vi "SPWB_Create.vi"(0 "reference in":refnum<class "SPWB.lvclass">, 5 "error in (no error)":errorcluster, 6 "Version #":string, 7 "Application Name":string, 9 "Window Name Index":string, 11 "State Queue":string[](array[string])) -> (14 "reference out":refnum<class "SPWB.lvclass">, 19 "error out":errorcluster)   [LabVIEW 2022 SP3, in "SPWB.lvclass"]
doc: "Constructor."
uses:
  SPWB.lvclass
  C:/Program Files/National Instruments/LabVIEW 2022/vi.lib/addons/_AddQ/G#Object/G#Object.lvclass
  W:/projects/archives/23 Charette AI Group/SPWB/API/Generic Utilities_class/Generic Utilities.lvclass
  API/Registration_class/utils/Registration Type.ctl
  <vilib>/addons/_AddQ/G#Object/G#Object.lvclass
  API/GSwFormDSP_class/GSwFormDSP.lvclass
  API/Generic Utilities_class/Generic Utilities.lvclass
  API/Registration_class/Registration.lvclass
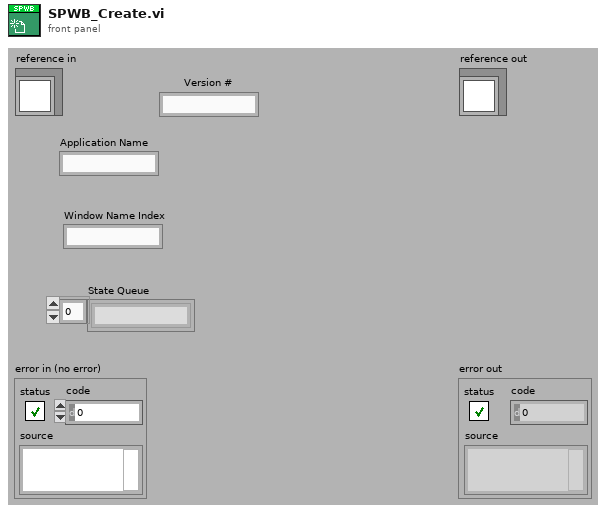
[diagram p1: front panel]
types:
  T1 = typedef "Registration.lvclass/Registration Type.ctl" = enum16{"Unregistered", "Registered - Full Activation", "Not Required- Full Activation"}
  T2 = typedef "SPWB.lvclass/ObjectAttributesRef.ctl" = refnum<data-value>
  T3 = typedef "SPWB.lvclass/ObjectAttributes.ctl" = cluster{"Window Name Index":string, "Data":refnum<class "GSwFormDSP.lvclass">, "Registration":refnum<class "Registration.lvclass">, "TFA User Control Refs ":T4}
  T4 = typedef "SPWB.lvclass/TFA - User Control References.ctl" = cluster{"STFT Graph":refnum<vi>, "Time Section":refnum<vi>, "Frequency Section":refnum<vi>}
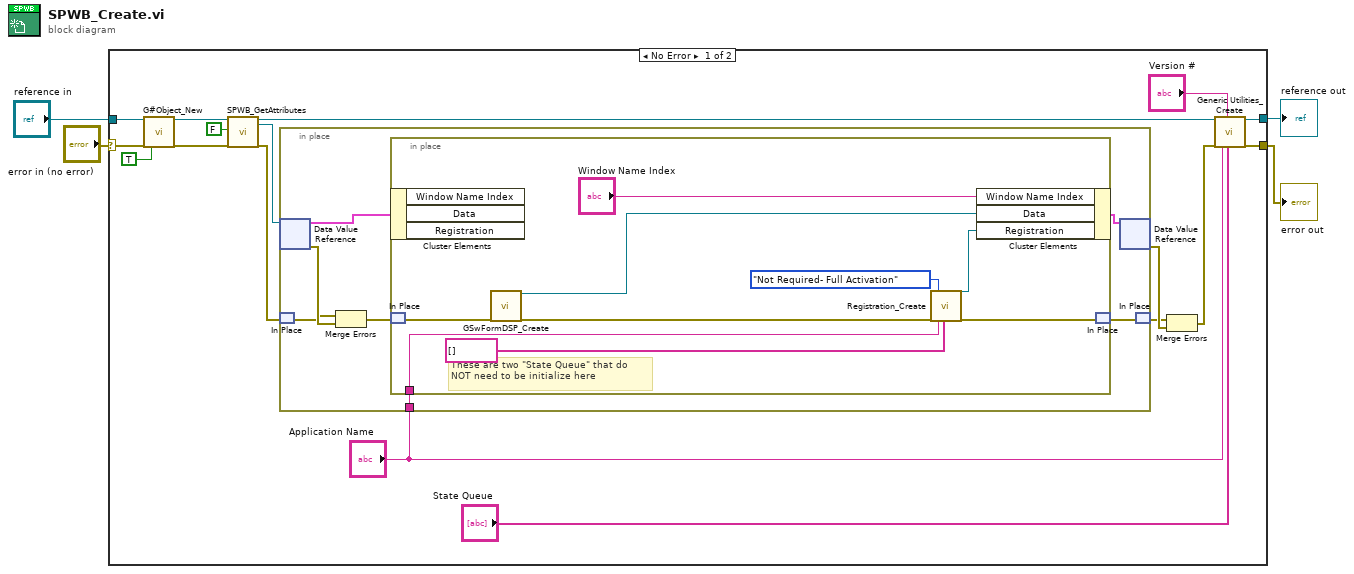
[diagram p0: block diagram]
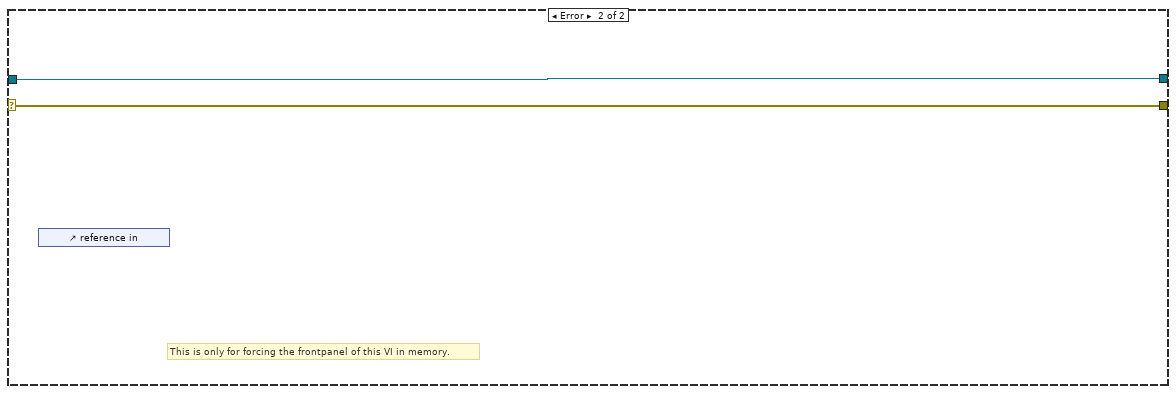
[diagram p2: hidden frame]
diagram:
  n1 = case shown="No Error" "error in (no error)" {
    selector: "error in (no error)" -> [w20 w39]
    tunnel: [w10 w39] -> w3
    tunnel: [w12 w38] -> w1
    tunnel: "reference in" -> [w21 w38]
    frame No Error {
      n2 = call <vilib>:"G#Object_New.vi"("reference in"=w21, "error in (no error)"=w20, "user counter (T)?"=TRUE ("User Counter")) -> ("reference out"=w15:refnum<class "SPWB.lvclass">, "error out"=w14:errorcluster)  [unwired: 14 in, 1 out]
      n3 = call "SPWB_GetAttributes.vi"("reference in"=w15, "return data? (T)"=FALSE ("return data"), "error in (no error)"=w14) -> ("reference out"=w13:refnum<class "SPWB.lvclass">, "attributes ref"=w17:T2, "error out"=w7:errorcluster)  [unwired: 13 in, 1 out]
      n4 = in-place {
        in-place-border: "Application Name" -> [w26]
        n5 = in-place-dvr #1(w17) -> (w27:T3, w25:errorcluster)
        n6 = in-place-match #2(w7) -> (w24:errorcluster)
        n7 = Merge Errors(w24, w25) -> (w23:errorcluster)
        n8 = in-place {
          in-place-border: w26 -> [w34]
          # "These are two \"State Queue\" that do NOT need to be initialize here"
          n9 = in-place-cluster #3(w27) -> ()  [unwired: 3 out]
          n10 = in-place-match #4(w23) -> (w31:errorcluster)
          n11 = call "GSwFormDSP_Create.vi"("error in (no error)"=w31) -> ("reference out"=w36:refnum<class "GSwFormDSP.lvclass">, "error out"=w35:errorcluster)  [unwired: 17 in]
          n12 = call "Registration_Create.vi"("error in (no error)"=w35, "Registration Level"=Registration_Type."Not Required- Full Activation", "Application Name"=w34, "State Queue"=string[] []) -> ("reference out"=w32:refnum<class "Registration.lvclass">, "error out"=w30:errorcluster)  [unwired: 14 in]
          n13 = in-place-cluster #3("Window Name Index"="Window Name Index", "Data"=w36, "Registration"=w32) -> (w28:T3)
          n14 = in-place-match #4(w30) -> (w22:errorcluster)
        }
        n15 = in-place-dvr #1(w28) -> (w18:errorcluster)  [unwired: 1 out]
        n16 = in-place-match #2(w22) -> (w6:errorcluster)
      }
      n17 = Merge Errors(w6, w18) -> (w11:errorcluster)
      n18 = call "Generic Utilities_Create.vi"("reference in"=w13, "error in (no error)"=w11, "Application Name"="Application Name", "Version #"="Version #", "State Queue"="State Queue") -> ("reference out"=w12:refnum<class "SPWB.lvclass">, "error out"=w10:errorcluster)  [unwired: 13 in]
    }
    frame Error {
      # "This is only for forcing the frontpanel of this VI in memory."
      n19 = control-ref of="reference in"() -> ()  [unwired: 1 out]
    }
  }
  "error out" <- w3
  "reference out" <- w1
